vi "Create Items From Spreadsheet.vi"(8 "error in (no error)":errorcluster, 10 "file path (use dialog)":path, 11 "Custom Device in":refnum<k24>) -> (0 "error out":errorcluster, 2 "Channel Created Inside NIVS Address Range":bool[](array[boolean]), 3 "Custom Device out":refnum<k24>)   [LabVIEW 2010, in "RefMem PtByPt System Definition API.lvlib"]
doc: "Set the VISA name and Decimation of the custom device."
uses:
  RefMem PtByPt System Definition API.lvlib
  NationalInstruments.VeriStand.SystemDefinitionAPI
  Custom Device/RefMem PtByPt Custom Device.lvlib
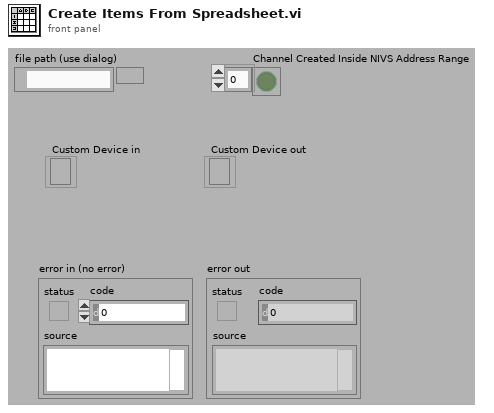
[diagram p1: front panel]
types:
  T1 = typedef "Custom Device API.lvlib/Custom Device Pointer.ctl" = refnum<k24>
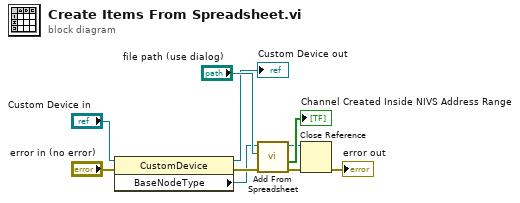
[diagram p0: block diagram]
diagram:
  n1 = property class="CustomDevice"(reference="Custom Device in", error in="error in (no error)") -> (reference out=→"Custom Device out":refnum<k24>, error out=w7:errorcluster, "BaseNodeType"=w5:refnum<k24>)
  n2 = call "Add From Spreadsheet.vi"("error in (no error)"=w7, "file path (use dialog)"="file path (use dialog)", "Device BaseNodeType in"=w5) -> ("error out"=w3:errorcluster, "Address warning"=→"Channel Created Inside NIVS Address Range":bool[], "Device BaseNodeType out"=w2:T1)  [unwired: 6 in]
  n3 = Close Reference(reference=w2, error in (no error)=w3) -> (error out=→"error out":errorcluster)
